vi "Motor_Experiment.vi"() -> ()   [LabVIEW 2017]
uses:
  <vilib>/myRIO/Instrument Drivers/Onboard IO/DIO/typedefs/DIO Reference.ctl
  <vilib>/myRIO/Common/Instrument Driver Framework/Utilities/typedefs/myRIO Generic Hardware Reference.ctl
  <vilib>/myRIO/Common/Instrument Driver Framework/Utilities/typedefs/Hardware Version Enum.ctl
  <vilib>/myRIO/Common/Instrument Driver Framework/Utilities/typedefs/myRIO v1.0 Reference.ctl
  <vilib>/myRIO/Common/Instrument Driver Framework/Utilities/typedefs/Generic FPGA Reference.ctl
  <vilib>/myRIO/Common/Instrument Driver Framework/myRIO v1.0/DIO/typedefs/DIO Channels List.ctl
  <vilib>/myRIO/Common/Instrument Driver Framework/myRIO v1.0/DIO/typedefs/DIO Channels Enum.ctl
  <vilib>/userdefined/High Color/nirio_resource_hc.ctl
  <vilib>/myRIO/Common/Instrument Driver Framework/myRIO v1.0/Encoder/typedefs/Encoder Signal Mode.ctl
  <vilib>/myRIO/Instrument Drivers/Onboard IO/Encoder/typedefs/Encoder Reference.ctl
  <vilib>/myRIO/Common/Instrument Driver Framework/myRIO v1.0/Encoder/typedefs/Encoder Channels Enum.ctl
  <vilib>/myRIO/Common/Instrument Driver Framework/myRIO v1.0/Encoder/typedefs/Encoder Configuration v1.0.ctl
  <vilib>/myRIO/Instrument Drivers/Onboard IO/PWM/typedefs/PWM Reference.ctl
  <vilib>/myRIO/Common/Instrument Driver Framework/myRIO v1.0/PWM/typedefs/PWM Channels Enum.ctl
  <vilib>/myRIO/Instrument Drivers/Onboard IO/PWM/typedefs/PWM Configuration.ctl
  <vilib>/myRIO/Common/Instrument Driver Framework/Utilities/vis/Is FPGA Ref Available.vi
  <vilib>/myRIO/Common/Instrument Driver Framework/myRIO v1.0/DIO/vis/myRIO v1.1 Open DIO.vi
  <vilib>/myRIO/Instrument Drivers/Onboard IO/DIO/vis/Write.vi
  <vilib>/myRIO/Common/Instrument Driver Framework/myRIO v1.0/Encoder/vis/myRIO v1.1 Open Encoder.vi
  <vilib>/myRIO/Instrument Drivers/Onboard IO/Encoder/vis/Read.vi
  <vilib>/myRIO/Common/Instrument Driver Framework/myRIO v1.0/PWM/vis/myRIO v1.1 Open PWM.vi
  <vilib>/myRIO/Instrument Drivers/Onboard IO/PWM/vis/Set Duty Cycle and Frequency.vi
  <vilib>/myRIO/Common/Instrument Driver Framework/Utilities/vis/Validate Channels.vi
  <vilib>/myRIO/Common/Instrument Driver Framework/myRIO v1.0/DIO/vis/myRIO v1.0 Reserve DIO.vi
  <vilib>/myRIO/Common/Instrument Driver Framework/myRIO v1.0/Encoder/vis/myRIO v1.0 Reserve Encoder.vi
  <vilib>/myRIO/Common/Instrument Driver Framework/myRIO v1.0/PWM/vis/myRIO v1.0 Reserve PWM.vi
  <vilib>/myRIO/Common/Instrument Driver Framework/myRIO v1.0/UART/vis/myRIO v1.0 Close UART.vi
  <vilib>/myRIO/Common/Instrument Driver Framework/myRIO v1.0/Resource Manager/vis/myRIO v1.0 Reserve Channel List.vi
  <vilib>/myRIO/Common/Instrument Driver Framework/myRIO v1.0/DIO/vis/myRIO v1.0 Build MUX Configuration DIO.vi
  <vilib>/myRIO/Common/Instrument Driver Framework/myRIO v1.0/Encoder/vis/myRIO v1.0 Build MUX Configuration Encoder.vi
  <vilib>/myRIO/Common/Instrument Driver Framework/myRIO v1.0/PWM/vis/myRIO v1.0 Build MUX Configuration PWM.vi
  <vilib>/myRIO/Common/Instrument Driver Framework/myRIO v1.0/Resource Manager/vis/myRIO v1.0 Reserve Channel.vi
  <vilib>/myRIO/Common/Instrument Driver Framework/myRIO v1.0/Resource Manager/vis/myRIO v1.0 Unreserve Channel.vi
  <vilib>/myRIO/Common/Instrument Driver Framework/myRIO v1.0/Resource Manager/vis/myRIO v1.0 Create Configuration List.vi
  <vilib>/myRIO/Common/Instrument Driver Framework/myRIO v1.0/Resource Manager/vis/myRIO v1.0 Build Mutex Name.vi
  <vilib>/Utility/VariantDataType/GetNumericInfo.vi
  <vilib>/Utility/error.llb/Error Cluster From Error Code.vi
  <vilib>/myRIO/Common/Instrument Driver Framework/myRIO v1.0/myRIO v1.1 Open.vi
  <vilib>/myRIO/Common/Instrument Driver Framework/Utilities/vis/IO Manager.vi
  <vilib>/myRIO/Common/Instrument Driver Framework/Utilities/vis/Configuration Manager.vi
  <vilib>/myRIO/Common/Instrument Driver Framework/myRIO v1.0/Resource Manager/vis/myRIO v1.0 Configure IO.vi
  <vilib>/myRIO/Common/Instrument Driver Framework/myRIO v1.0/myRIO v1.0 Close.vi
  <vilib>/myRIO/Common/Instrument Driver Framework/myRIO v1.0/DIO/vis/myRIO v1.0 Write DIO.vi
  <vilib>/myRIO/Common/Instrument Driver Framework/myRIO v1.0/Encoder/vis/myRIO v1.0 Configure Encoder.vi
  <vilib>/myRIO/Common/Instrument Driver Framework/myRIO v1.0/Encoder/vis/myRIO v1.0 Read Encoder.vi
  <vilib>/myRIO/Common/Instrument Driver Framework/myRIO v1.0/PWM/vis/myRIO v1.0 Write PWM.vi
  <vilib>/myRIO/Common/Instrument Driver Framework/Utilities/vis/FPGA Ref Manager.vi
  <vilib>/myRIO/Common/Instrument Driver Framework/myRIO v1.0/myRIO v1.0 Reset FPGA.vi
  <vilib>/myRIO/Common/Instrument Driver Framework/myRIO v1.0/IRQ/vis/myRIO v1.0 IRQ Info FGV.vi
  <vilib>/myRIO/Common/Instrument Driver Framework/myRIO v1.0/IRQ/vis/myRIO v1.0 Timer IRQ Info FGV.vi
  <vilib>/myRIO/Common/Instrument Driver Framework/myRIO v1.0/IRQ/vis/myRIO v1.0 ISR Agent.vi
  <vilib>/myRIO/Express VI/Onboard IO/DO/DO Express VI.xnode
  <vilib>/myRIO/Instrument Drivers/Onboard IO/DIO/vis/myRIO DIO Open.xnode
  <vilib>/myRIO/Express VI/Onboard IO/Encoder/Encoder Express VI.xnode
  <vilib>/myRIO/Instrument Drivers/Onboard IO/Encoder/vis/myRIO Encoder Open.xnode
  <vilib>/myRIO/Common/Instrument Driver Framework/myRIO v1.0/Encoder/typedefs/Encoder Count Direction Enum.ctl
  <vilib>/myRIO/Express VI/Onboard IO/PWM/PWM Express VI.xnode
  <vilib>/myRIO/Instrument Drivers/Onboard IO/PWM/vis/myRIO PWM Open.xnode
  <vilib>/myRIO/Instrument Drivers/Utilities/Utilities.lvlib
  <vilib>/myRIO/Instrument Drivers/Onboard IO/PWM/PWM.lvlib
  <vilib>/myRIO/Instrument Drivers/Onboard IO/DIO/DIO.lvlib
  <vilib>/myRIO/Instrument Drivers/Onboard IO/Encoder/Encoder.lvlib
panel:
  out "Signals":dbl[][](graph)
  in  "Direction":bool=TRUE
  in  "Start Experiment":bool
  out "Numeric":dbl
  in  "Acceleration time (ms)":dbl
  in  "STOP":bool
  out "error out":errorcluster
  # "Nota: NUNCA PARE EL PROGARMA CON EL BOTON DE ABORTAR. \nPASE LO QUE PASE; DETENER EL PROGARMA CON ESTE BOTON STOP"
  # "Backward"
  # "Forward"
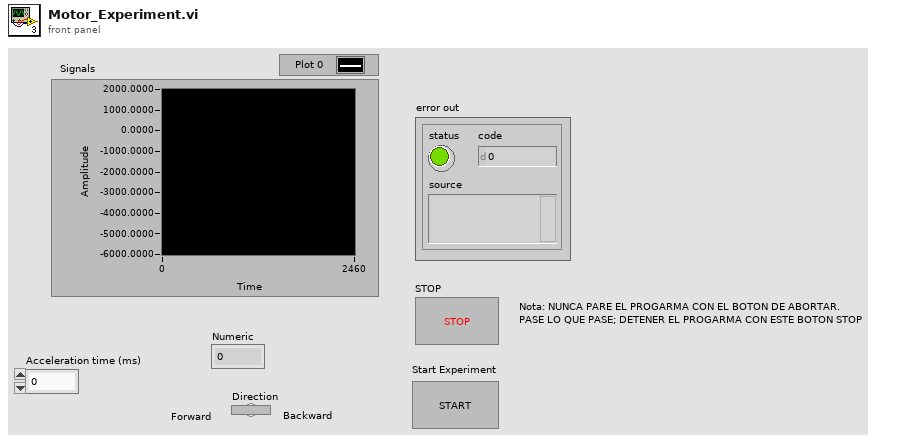
[diagram p1: front panel]
types:
  T1 = enum16{"Default", "Accelerate", "Constant", "Decelerate", "Fin"}
  T2 = typedef "Encoder.lvlib/Encoder Reference.ctl" = cluster{"myRIO Reference":T3, "Encoder Channels Enum":T7}
  T3 = typedef "myRIO Generic Hardware Reference.ctl" = cluster{"myRIO Model":T4, "myRIO Hardware Reference":T5}
  T4 = typedef "Hardware Version Enum.ctl" = enum16{"Unknown", "myRIO-1900", "myRIO-1950", "roboRIO", "NI ELVIS RIO CM"}
  T5 = typedef "myRIO v1.0 Reference.ctl" = cluster{"Generic FPGA Reference":T6, "Allow multiple opens":bool}
  T6 = typedef "Generic FPGA Reference.ctl" = refnum<k20>
  T7 = typedef "Encoder Channels Enum.ctl" = enum16{"Not Connected", "C/ENC0", "C/ENC1", "A/ENC", "B/ENC", "DIO/ENC0", "DIO/ENC1", "DIO/ENC2", "DIO/ENC3", "DIO/ENC4"}
  T8 = typedef "Encoder Signal Mode.ctl" = enum16{"Quadrature phase signal", "Step and direction signal"}
  T9 = typedef "nirio_resource_hc.ctl" = tag
  T10 = typedef "PWM.lvlib/PWM Reference.ctl" = cluster{"myRIO Reference":T3, "PWM Channels Enum":T11, "PWM Configuration":T12}
  T11 = typedef "PWM Channels Enum.ctl" = enum16{"Not Connected", "C/PWM0", "C/PWM1", "A/PWM0", "A/PWM1", "A/PWM2", "B/PWM0", "B/PWM1", "B/PWM2", "PWM/PWM0", "PWM/PWM1", "PWM/PWM2", "PWM/PWM3", "PWM/PWM4", "PWM/PWM5", "PWM/PWM6", "PWM/PWM7", "PWM/PWM8", "PWM/PWM9"}
  T12 = typedef "PWM.lvlib/PWM Configuration.ctl" = cluster{"Frequency":dbl, "Duty Cycle":dbl}
  T13 = typedef "DIO.lvlib/DIO Reference.ctl" = cluster{"myRIO Reference":T3, "DIO Channels List":T14}
  T14 = typedef "DIO Channels List.ctl" = T15[]
  T15 = typedef "DIO Channels Enum.ctl" = enum16{"Not Connected", "C/DIO0", "C/DIO1", "C/DIO2", "C/DIO3", "C/DIO4", "C/DIO5", "C/DIO6", "C/DIO7", "A/DIO0", "A/DIO1", "A/DIO2", "A/DIO3", "A/DIO4", "A/DIO5", "A/DIO6", "A/DIO7", "A/DIO8", "A/DIO9", "A/DIO10", "A/DIO11", "A/DIO12", "A/DIO13", "A/DIO14", "A/DIO15", "B/DIO0", "B/DIO1", "B/DIO2", "B/DIO3", "B/DIO4", "B/DIO5", "B/DIO6", "B/DIO7", "B/DIO8", "B/DIO9", "B/DIO10", "B/DIO11", "B/DIO12", "B/DIO13", "B/DIO14", "B/DIO15", "LED0", "LED1", "LED2", "LED3", "Button0", "DIO/DIO0", "DIO/DIO1", "DIO/DIO2", "DIO/DIO3", "DIO/DIO4", "DIO/DIO5", "DIO/DIO6", "DIO/DIO7", "DIO/DIO8", "DIO/DIO9", "SPI/CS0", "SPI/CS1", "SPI/CS2", "SPI/CS3", "LED RADIO (Green)", "LED RADIO (Red)", "LED COMM (Green)", "LED COMM (Red)", "LED MODE (Green)", "LED MODE (Red)"}
  T16 = enum16{"Default", "Accelerate", "Constant", "Decelerate"}
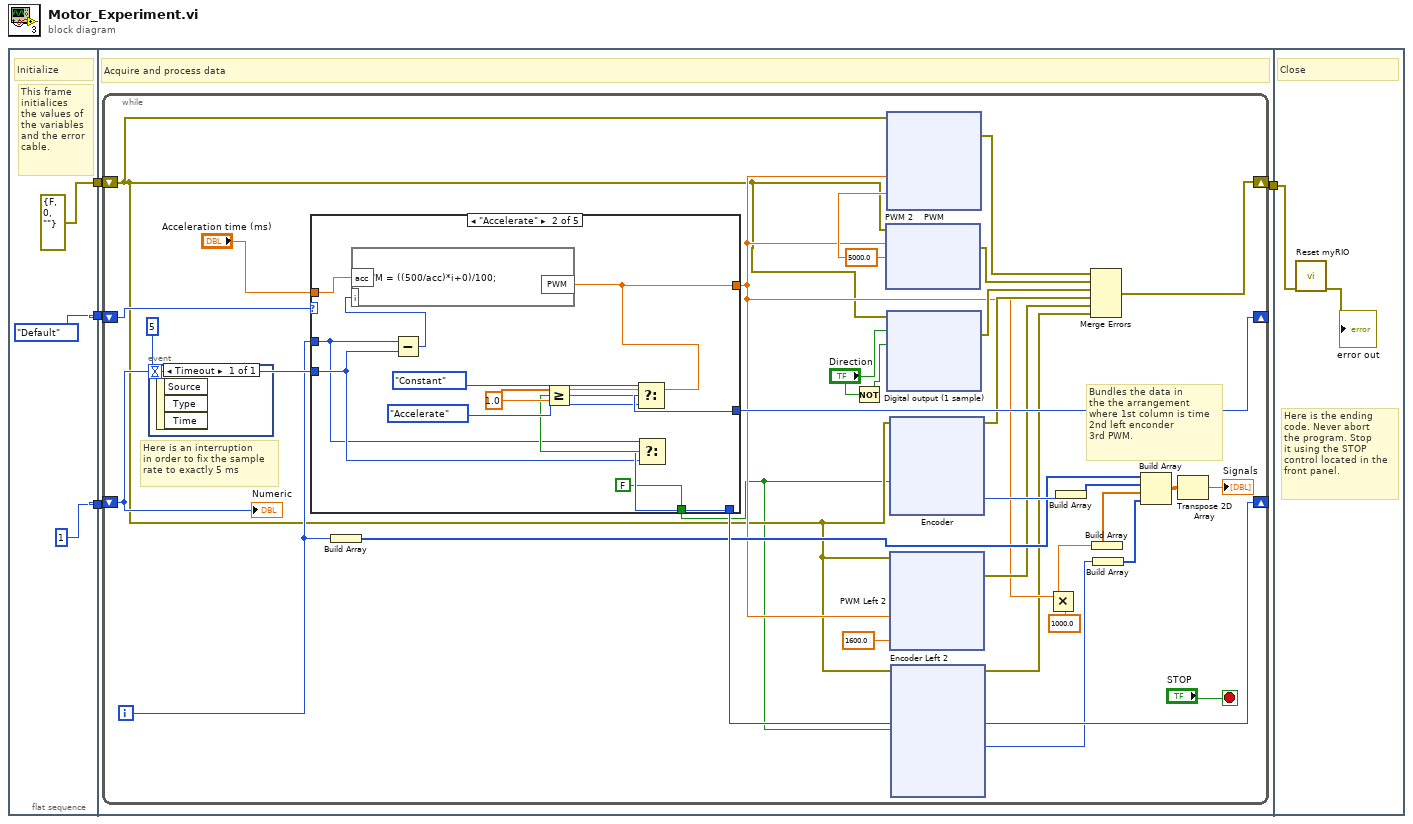
[diagram p0: block diagram]
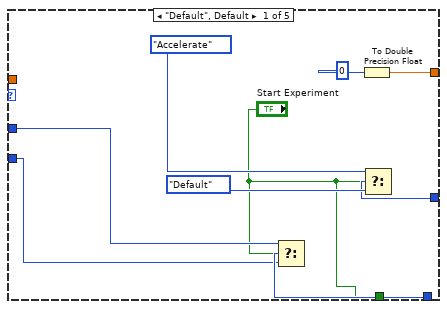
[diagram p2: hidden frame]
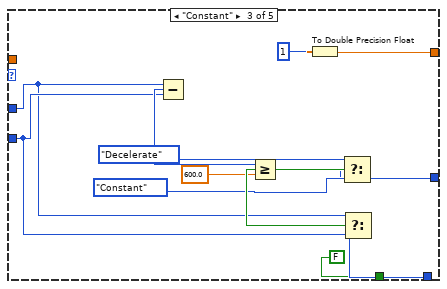
[diagram p3: hidden frame]
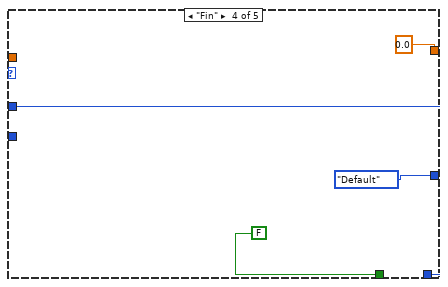
[diagram p4: hidden frame]
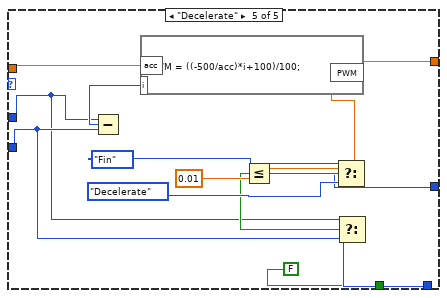
[diagram p5: hidden frame]
diagram:
  n1 = flat-sequence {
    tunnel: [errorcluster {"status"=FALSE, "code"=0, "source"=""} ("error in (no error)")] -> w4
    tunnel: [T1."Default"] -> w3
    tunnel: [1] -> w2
    tunnel: w4 -> [w9]
    tunnel: w3 -> [w11]
    tunnel: w2 -> [w10]
    tunnel: [w8] -> w1
    tunnel: w1 -> [w326]
    frame #0 {
      # "This frame \ninitialices\nthe values of\nthe variables\nand the error \ncable."
      # "Initialize"
    }
    frame #1 {
      # "Acquire and process data"
      n2 = while {
        shift-right: [w41] -> _
        shift-left: w10 -> [w40]
        shift-right: [w42] -> _
        shift-left: w11 -> [w39]
        shift-right: [w29] -> w8
        shift-left: w9 -> [w17]
        i -> [w27]
        stop <- "STOP" stop-if-true
        w37 = 5000.0 ("Frequency [Hz]")
        # "Bundles the data in \nthe the arrangement\nwhere 1st column is time\n2nd left enconder\n3rd PWM."
        # "Here is an interruption\nin order to fix the sample \nrate to exactly 5 ms"
        n3 = event shown="[0] Timeout" {
          selector: _ -> [_]
          dyn-events: _ -> [_]
          timeout: 5 -> [_]
          event Timeout {
            n4 = event-data() -> ()  [unwired: 1 in, 3 out]
          }
        }
        n5 = case shown="\"Accelerate\"" w39 {
          tunnel: w40 -> [w278 w288 w300 _ w317]
          tunnel: "Acceleration time (ms)" -> [_ w297 _ _ w321]
          tunnel: [w284 w295 w303 0.0 ("PWM") w320] -> w18
          tunnel: [w281 w293 w305 T1."Default" w319] -> w42
          tunnel: [w280 w289 w304 w312 w318] -> w41
          tunnel: w27 -> [w279 w287 w299 w312 w316]
          tunnel: ["Start Experiment" FALSE FALSE FALSE FALSE] -> w12
          frame "Default", Default {
            n6 = Select(t=w279, s="Start Experiment", f=w278) -> (s? t:f=w280:i32)
            n7 = To Double Precision Float(number=0) -> (double precision float=w284:dbl)
            n8 = Select(t=T1."Accelerate", s="Start Experiment", f=T1."Default") -> (s? t:f=w281:T1)
          }
          frame "Accelerate" {
            n9 = Subtract(x=w287, y=w288) -> (x-y=w291:i32)
            n10 = formula code="PWM = ((500/acc)*i+0)/100;"("acc"=w297, "i"=w291) -> ("PWM"=w295:dbl)
            n11 = Greater Or Equal?(x=w295, y=1.0) -> (x >= y?=w290:bool)
            n12 = Select(t=T16."Constant", s=w290, f=T16."Accelerate") -> (s? t:f=w293:T16)
            n13 = Select(t=w287, s=w290, f=w288) -> (s? t:f=w289:i32)
          }
          frame "Constant" {
            n14 = Subtract(x=w299, y=w300) -> (x-y=w301:i32)
            n15 = Greater Or Equal?(x=w301, y=600.0) -> (x >= y?=w309:bool)
            n16 = To Double Precision Float(number=1) -> (double precision float=w303:dbl)
            n17 = Select(t=T16."Decelerate", s=w309, f=T16."Constant") -> (s? t:f=w305:T16)
            n18 = Select(t=w299, s=w309, f=w300) -> (s? t:f=w304:i32)
          }
          frame "Fin" {
          }
          frame "Decelerate" {
            n19 = Subtract(x=w316, y=w317) -> (x-y=w323:i32)
            n20 = formula code="PWM = ((-500/acc)*i+100)/100;"("acc"=w321, "i"=w323) -> ("PWM"=w320:dbl)
            n21 = Less Or Equal?(x=w320, y=0.01) -> (x <= y?=w322:bool)
            n22 = Select(t=T1."Fin", s=w322, f=T16."Decelerate") -> (s? t:f=w319:T1)
            n23 = Select(t=w316, s=w322, f=w317) -> (s? t:f=w318:i32)
          }
        }
        n24 = Build Array(w27) -> (w26:i32[])
        n25 = Not(x="Direction") -> (.not. x?=w33:bool)
        n26 = xnode "PWM 2"("error in (no error)"=w17, "Duty Cycle"=w18, "Frequency [Hz]"=w37) -> ("error out"=w35:errorcluster)
        n27 = xnode "PWM"("Duty Cycle"=w18, "Frequency [Hz]"=w37, "error in (no error)"=w17) -> ("error out"=w36:errorcluster)
        n28 = xnode "Digital output (1 sample)"("error in (no error)"=w17, "A/DIO3 (Pin 17)"="Direction", "A/DIO2 (Pin 15)"=w33) -> ("error out"=w34:errorcluster)
        n29 = xnode "Encoder"("Reset Counter"=w12, "error in (no error)"=w17) -> ("Counter Value"=w28:i32, "error out"=w31:errorcluster)  [unwired: 2 out]
        n30 = xnode "PWM Left 2"("Duty Cycle"=w18, "Frequency [Hz]"=1600.0, "error in (no error)"=w17) -> ("error out"=w20:errorcluster)
        n31 = xnode "Encoder Left 2"("Reset Counter"=w12, "error in (no error)"=w17) -> ("Counter Value"=w13:i32, "error out"=w16:errorcluster)  [unwired: 2 out]
        n32 = Multiply(x=w18, y=1000.0) -> (x*y=w21:dbl)
        n33 = Build Array(w28) -> (w25:i32[])
        n34 = Merge Errors(w36, w35, w34, w31, w20, w16) -> (w29:errorcluster)
        n35 = Build Array(w21) -> (w15:dbl[])
        n36 = Build Array(w13) -> (w14:i32[])
        n37 = Build Array(w26, w25, w15, w14) -> (w24:dbl[][])
        n38 = Transpose 2D Array(2D array=w24) -> (transposed array=→"Signals":dbl[][])
        "Numeric" <- w40
      }
    }
    frame #2 {
      # "Here is the ending \ncode. Never abort \nthe program. Stop\nit using the STOP \ncontrol located in the\nfront panel."
      # "Close"
      n39 = call <vilib>:"Reset myRIO.vi"("error in (no error)"=w326) -> ("error out"=→"error out":errorcluster)  [unwired: 10 in]
    }
  }
